vi "__Init Local List Menu.vi"(8 "error in (no error)":errorcluster, 9 "MCListbox Refnum":refnum<vi>, 10 "Coords":T1, 11 "menu reference":refnum<k9>) -> (0 "error out":errorcluster, 3 "Discard?":bool)   [LabVIEW 2011]
doc: "Fills the right-click menu associated with the local list Multicolumn Listbox with the proper items, based on what kind of item the click happened on (file/folder/empty item)."
uses:
  <vilib>/Utility/miscctls.llb/LVPoint32TypeDef.ctl
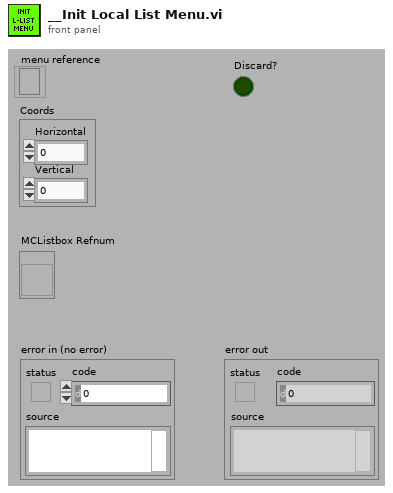
[diagram p1: front panel]
types:
  T1 = typedef "LVPoint32TypeDef.ctl" = cluster{"Horizontal":i32, "Vertical":i32}
  T2 = typedef "LVRowAndColumnTypeDef.ctl" = cluster{"Row":i32, "Column":i32}
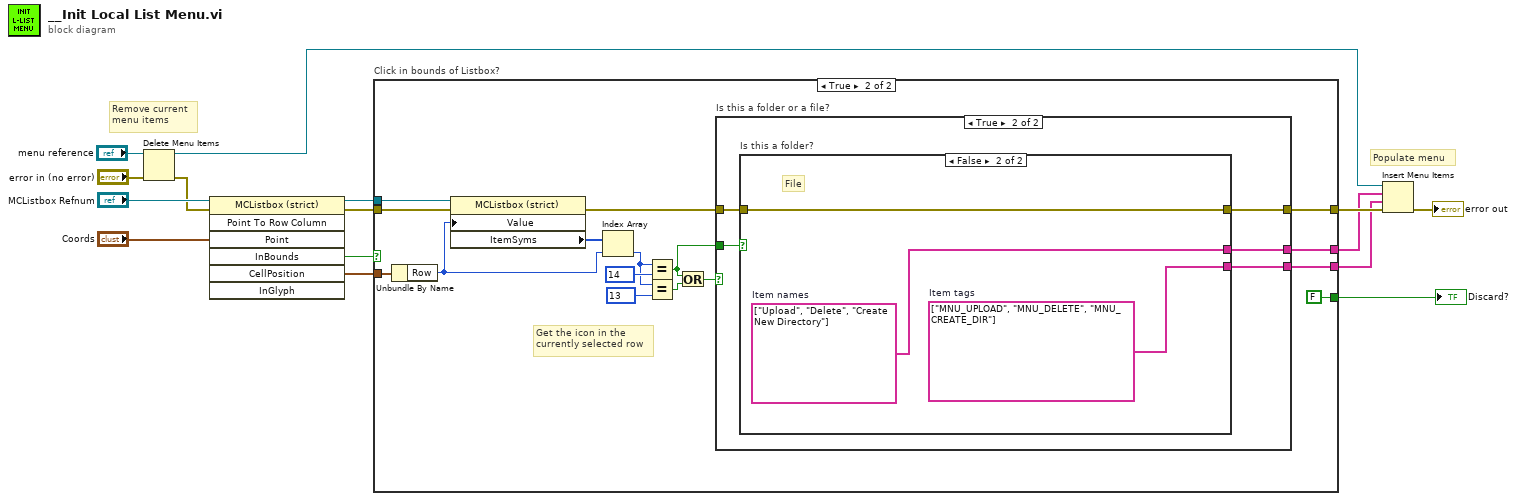
[diagram p0: block diagram]
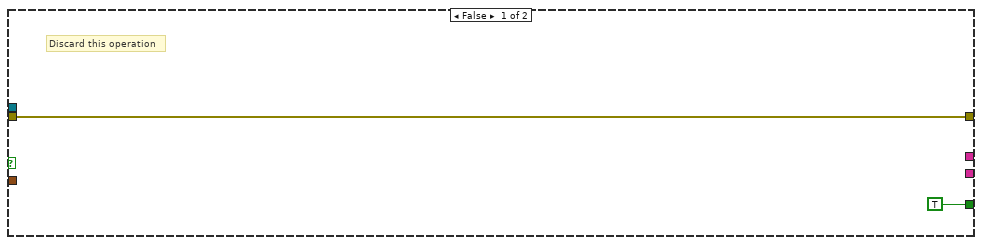
[diagram p2: hidden frame]
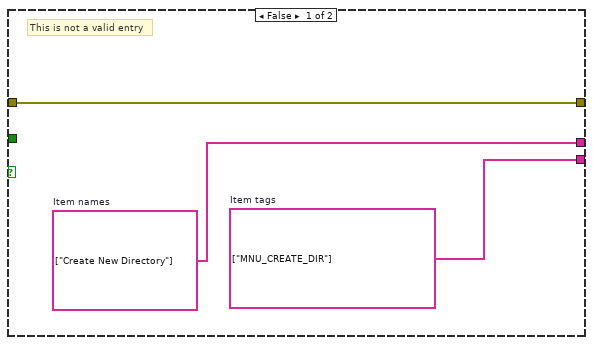
[diagram p3: hidden frame]
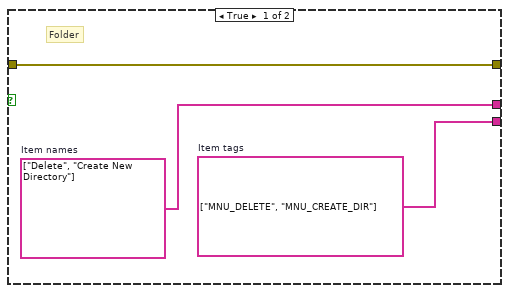
[diagram p4: hidden frame]
diagram:
  # "Populate menu"
  # "Remove current\nmenu items"
  n1 = Delete Menu Items(6:"error in (no error)", 9:"menu reference") -> (0:w11:errorcluster, 3:w3:refnum<k9>)  [unwired: 2 in]
  n2 = invoke class="MCListbox (strict)" method="Point To Row Column"(reference="MCListbox Refnum", error in=w11, "Point"="Coords") -> (reference out=w7:refnum<vi>, error out=w8:errorcluster, "InBounds"=w10:bool, "CellPosition"=w9:T2)  [unwired: 4 in, 3 out]
  n3 = case "Click in bounds of Listbox?" shown="True" w10 {
    tunnel: w9 -> [_ w33]
    tunnel: w8 -> [w17 w32]
    tunnel: w7 -> [_ w31]
    tunnel: [_ w23] -> w5
    tunnel: [_ w22] -> w4
    tunnel: [w17 w20] -> w6
    tunnel: [TRUE FALSE] -> w1
    frame False {
      # "Discard this operation"
    }
    frame True {
      # "Get the icon in the\ncurrently selected row"
      n4 = Unbundle By Name(w33) -> ("Row"=w29:i32)
      n5 = property class="MCListbox (strict)"(reference=w31, error in=w32, "Value"=w29) -> (error out=w21:errorcluster, "ItemSyms"=w30:i32[])  [unwired: 1 out]
      n6 = Index Array(array=w30, index=w29) -> (element=w26:i32)
      n7 = Equal?(x=w26, y=14) -> (x = y?=w18:bool)
      n8 = Equal?(x=w26, y=13) -> (x = y?=w25:bool)
      n9 = Or(x=w18, y=w25) -> (x .or. y?=w24:bool)
      n10 = case "Is this a folder or a file?" shown="True" w24 {
        tunnel: [w35 w41] -> w23
        tunnel: [w34 w40] -> w22
        tunnel: w21 -> [w36 w39]
        tunnel: [w36 w38] -> w20
        tunnel: w18 -> [_ w37]
        frame False {
          w34 = string[] ["MNU_CREATE_DIR"]  # Item tags
          w35 = string[] ["Create New Directory"]  # Item names
          # "This is not a valid entry"
        }
        frame True {
          n11 = case "Is this a folder?" shown="False" w37 {
            tunnel: [w44 w47] -> w41
            tunnel: [w43 w46] -> w40
            tunnel: w39 -> [w42 w45]
            tunnel: [w42 w45] -> w38
            frame True {
              w43 = string[] ["MNU_DELETE", "MNU_CREATE_DIR"]  # Item tags
              w44 = string[] ["Delete", "Create New Directory"]  # Item names
              # "Folder"
            }
            frame False {
              w46 = string[] ["MNU_UPLOAD", "MNU_DELETE", "MNU_CREATE_DIR"]  # Item tags
              w47 = string[] ["Upload", "Delete", "Create New Directory"]  # Item names
              # "File"
            }
          }
        }
      }
    }
  }
  "Discard?" <- w1
  n12 = Insert Menu Items(6:w6, 7:w4, 8:w5, 9:w3) -> (0:→"error out":errorcluster)  [unwired: 2 in, 2 out]
